vi "Configure Timebase.vi"(8 "error in (no error)":errorcluster, 10 "Acquisition Time (50 ms)":dbl(ring)=0.05 items=["0.5m"=0.0005, "1m"=0.001, "2m"=0.002, "5m"=0.005, "10m"=0.01, "20m"=0.02, "50m"=0.05, "100m"=0.1, "200m"=0.2, "500m"=0.5], 11 "VISA resource name":refnum<visa-resource-name>) -> (0 "error out":errorcluster, 3 "VISA resource name out":refnum<visa-resource-name>)   [LabVIEW 2021, in "Yokogawa WT1800 Series.lvlib"]
doc: "Configures the timebase features."
uses:
  <instrlib>/Yokogawa WT1800 Series/Yokogawa WT1800 Series.lvlib
panel:
  # "s"
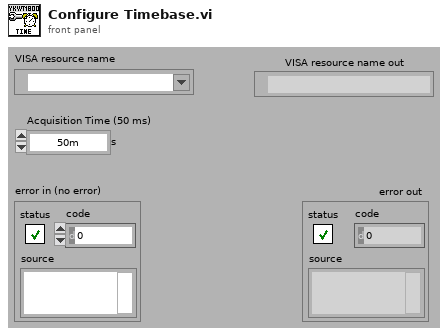
[diagram p1: front panel]
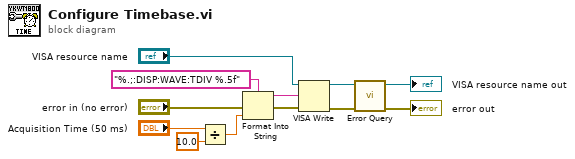
[diagram p0: block diagram]
diagram:
  n1 = Divide(x="Acquisition Time (50 ms)", y=10.0) -> (x/y=w3:dbl)
  n2 = Format Into String(format string="%.;:DISP:WAVE:TDIV %.5f" ("形式文字列"), error in="error in (no error)", w3) -> (resulting string=w6:string, error out=w4:errorcluster)  [unwired: 1 in]
  n3 = VISA Write ("VISA書き込み")(VISA resource name="VISA resource name", write buffer=w6, error in (no error)=w4) -> (VISA resource name out=w12:refnum<visa-resource-name>, error out=w11:errorcluster)  [unwired: 1 out]
  n4 = call <instrlib>:"Error Query.vi"("error in (no error)"=w11, "VISA resource name"=w12) -> ("error out"=→"error out":errorcluster, "VISA resource name out"=→"VISA resource name out":refnum<visa-resource-name>)  [unwired: 6 in, 2 out]
